vi "Read Depth.vi"(8 "error in (no error)":errorcluster, 11 "Picture in":refnum<class "Picture.lvclass">) -> (0 "error out":errorcluster, 2 "Depth":i32 caption="Depth (odd int)", 3 "Picture out":refnum<class "Picture.lvclass">)   [LabVIEW 2018, in "Picture.lvclass"]
uses:
  Picture.lvclass
  Picture.lvclass/Picture.ctl
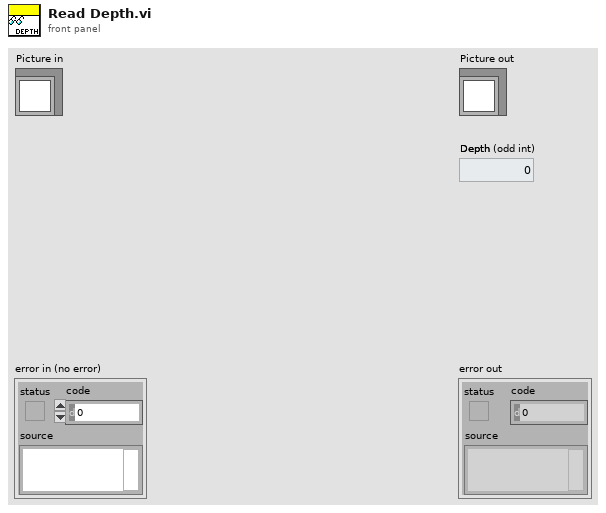
[diagram p1: front panel]
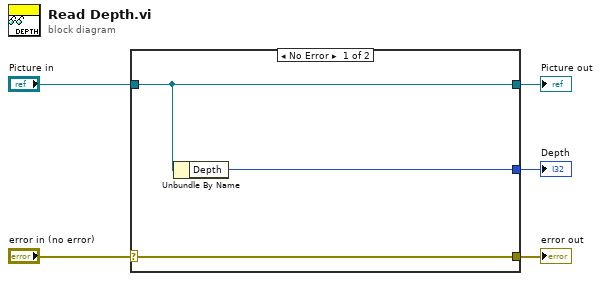
[diagram p0: block diagram]
diagram:
  n1 = case shown="No Error" "error in (no error)" {
    selector: "error in (no error)" -> [w8 w9]
    tunnel: [w8 w9] -> w4
    tunnel: [w7 w10] -> w2
    tunnel: "Picture in" -> [w7 w10]
    tunnel: [w6 _] -> w1
    frame No Error {
      n2 = Unbundle By Name(w7) -> ("Depth"=w6:i32)
    }
    frame Error {
    }
  }
  "error out" <- w4
  "Picture out" <- w2
  "Depth" <- w1
